vi "Adjust_ramp_rate.vi"(0 "Address":i32, 1 "VISA resource":refnum<visa-resource-name>, 2 "Ramp rate":dbl, 3 "error in":errorcluster, 4 "Control ramp":bool) -> (6 "error out":errorcluster)   [LabVIEW 2009]
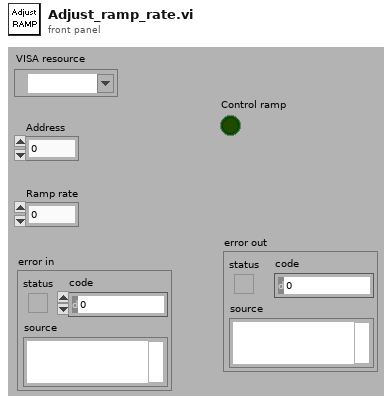
[diagram p1: front panel]
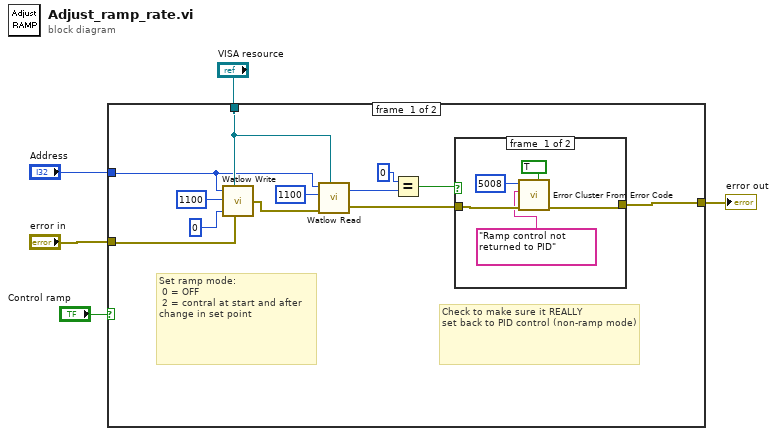
[diagram p0: block diagram]
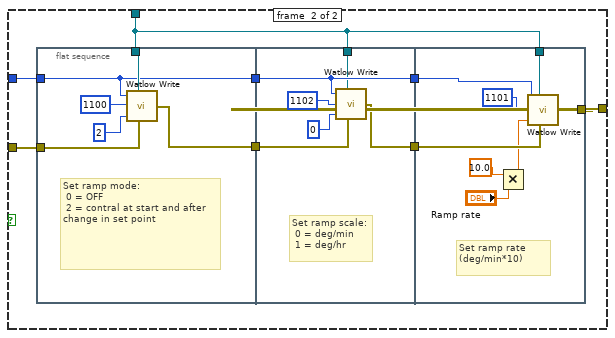
[diagram p3: hidden frame]
diagram:
  n1 = case shown="False" "Control ramp" {
    tunnel: "Address" -> [w11 w27]
    tunnel: "VISA resource" -> [w13 w24]
    tunnel: "error in" -> [w15 w26]
    tunnel: [w6 w25] -> w2
    frame #0 {
      # "Check to make sure it REALLY \nset back to PID control (non-ramp mode)"
      # "Set ramp mode:\n 0 = OFF\n 2 = contral at start and after change in set point"
      n2 = call "Watlow Write.vi"("Adress"=w11, "VISA resource name"=w13, "Register"=u32 1100, "Parameter"=u32 0, "error in (no error)"=w15) -> ("error out"=w14:errorcluster)
      n3 = call "Watlow Read.vi"("Adress"=w11, "Register"=u32 1100, "error in"=w14, "VISA resource name"=w13) -> ("Number"=w10:u32, "error out"=w7:errorcluster)  [unwired: 1 out]
      n4 = Equal?(x=u32 0, y=w10) -> (x = y?=w8:bool)
      n5 = case shown="False" w8 {
        tunnel: w7 -> [w22 w23]
        tunnel: [w18 w23] -> w6
        frame #0 {
          n6 = call <vilib>:"Error Cluster From Error Code.vi"("is warning? (False)"=TRUE, "error in (no error)"=w22, "error message (\"\")"="Ramp control not returned to PID", "error code (0)"=5008) -> ("error out"=w18:errorcluster)  [unwired: 1 in, 4 out]
        }
        frame #1 {
        }
      }
    }
    frame #1 {
      n7 = flat-sequence {
        tunnel: [w37] -> w31
        tunnel: w26 -> [w36]
        tunnel: w24 -> [w35]
        tunnel: w27 -> [w34]
        tunnel: [w34] -> w30
        tunnel: w31 -> [w43]
        tunnel: [w42] -> w29
        tunnel: w30 -> [w41]
        tunnel: [w41] -> w28
        tunnel: w24 -> [w38]
        tunnel: w29 -> [w51]
        tunnel: [w50] -> w25
        tunnel: w28 -> [w49]
        tunnel: w24 -> [w44]
        frame #0 {
          # "Set ramp mode:\n 0 = OFF\n 2 = contral at start and after change in set point"
          n8 = call "Watlow Write.vi"("Adress"=w34, "VISA resource name"=w35, "Register"=u32 1100, "Parameter"=u32 2, "error in (no error)"=w36) -> ("error out"=w37:errorcluster)
        }
        frame #1 {
          # "Set ramp scale:\n 0 = deg/min\n 1 = deg/hr"
          n9 = call "Watlow Write.vi"("Adress"=w41, "VISA resource name"=w38, "Register"=u32 1102, "Parameter"=u32 0, "error in (no error)"=w43) -> ("error out"=w42:errorcluster)
        }
        frame #2 {
          # "Set ramp rate\n(deg/min*10)"
          n10 = Multiply(x=10.0, y="Ramp rate") -> (x*y=w46:dbl)
          n11 = call "Watlow Write.vi"("Adress"=w49, "VISA resource name"=w44, "Register"=u32 1101, "Parameter"=w46, "error in (no error)"=w51) -> ("error out"=w50:errorcluster)
        }
      }
    }
  }
  "error out" <- w2
